vi "Publish Model Data.vi"(8 "error in (no error)":errorcluster, 9 "Data to Publish":variant, 10 "Topic Name":string, 11 "IModel in":refnum<class "IModel.lvclass">) -> (0 "error out":errorcluster, 3 "IModel out":refnum<class "IModel.lvclass">)   [LabVIEW 2015, in "IModel.lvlib" / "IModel.lvclass"]
uses:
  IModel.lvclass
  IModel.lvclass/IModel.ctl
  AbstractMessages/PreAddressedMsg/PreAddressedMsg.lvclass/PreAddressedMsg.ctl
  IMediator/IMediator Messages/Publish Msg/Publish Msg.lvclass/Publish Msg.ctl
  <vilib>/ActorFramework/Message Enqueuer/Message Enqueuer.lvclass/Message Enqueuer.ctl
  <vilib>/ActorFramework/Message Enqueuer/Enqueue.vi
  AbstractMessages/PreAddressedMsg/Read Return Address.vi
  <vilib>/ActorFramework/Message Priority Queue/Priority Enqueue.vi
  IMediator/IMediator Messages/Publish Msg/Publish Msg.lvclass
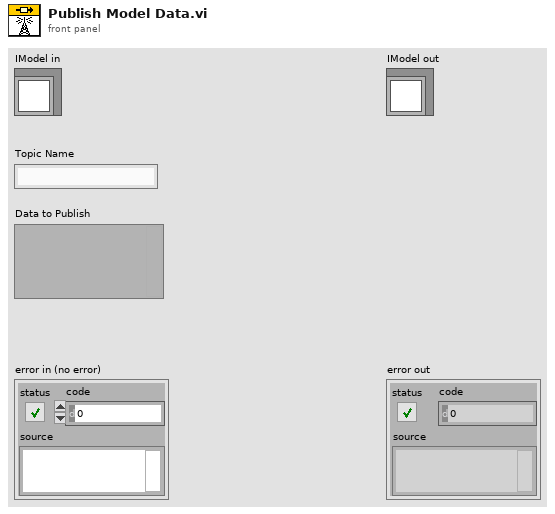
[diagram p1: front panel]
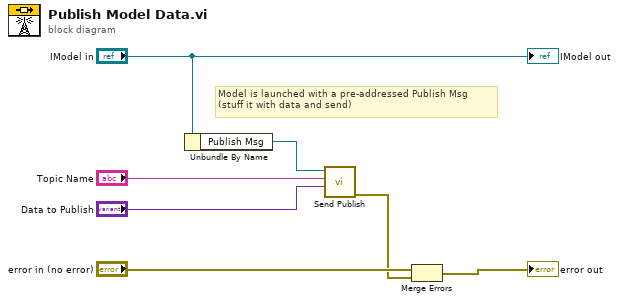
[diagram p0: block diagram]
diagram:
  # "Model is launched with a pre-addressed Publish Msg\n(stuff it with data and send)"
  n1 = Unbundle By Name("IModel in") -> ("Publish Msg"=w6:refnum<class "Publish Msg.lvclass">)
  n2 = call "Send Publish.vi"("Data to Publish"="Data to Publish", "Topic Name"="Topic Name", "Publish Message"=w6) -> ("error out"=w1:errorcluster)  [unwired: 7 in, 1 out]
  n3 = Merge Errors("error in (no error)", w1) -> (→"error out":errorcluster)
  "IModel out" <- "IModel in"
